vi "current measure.vi"(0 "VISA Refnum in":refnum<visa-resource-name>) -> (1 "read buffer":string, 2 "Numeric":dbl)   [LabVIEW 2025]
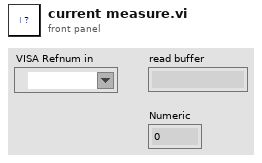
[diagram p1: front panel]
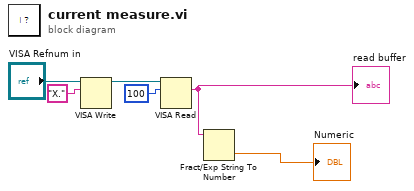
[diagram p0: block diagram]
diagram:
  n1 = VISA Write(VISA resource name="VISA Refnum in", write buffer="X.") -> (VISA resource name out=w1:refnum<visa-resource-name>)  [unwired: 1 in, 2 out]
  n2 = VISA Read(VISA resource name=w1, byte count=u32 100) -> (read buffer=w5:string)  [unwired: 1 in, 3 out]
  "read buffer" <- w5
  n3 = Fract/Exp String To Number(string=w5) -> (number=→"Numeric":dbl)  [unwired: 3 in, 1 out]
